vi "Create Missing Element.vi"(5 "Delimiter":string, 7 "Hierarchy":string[](array[string]), 10 "Element in":refnum<class "Config Element.lvclass">, 11 "Create":bool) -> (2 "Element":refnum<class "Config Element.lvclass">)   [LabVIEW 2020, in "CDM-Config.lvlib" / "Config Manager.lvclass"]
uses:
  Config Manager.lvclass
  Config Element/Config Element.lvclass
  <vilib>/AdvancedString/1D String Array to Delimited String.vi
  CDM-Config.lvlib
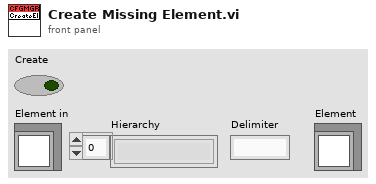
[diagram p1: front panel]
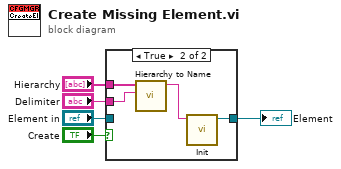
[diagram p0: block diagram]
diagram:
  n1 = case shown="True" "Create" {
    tunnel: "Element in" -> [w6 _]
    tunnel: [w6 w10] -> w3
    tunnel: "Delimiter" -> [_ w8]
    tunnel: "Hierarchy" -> [_ w9]
    frame False {
    }
    frame True {
      n2 = call "Hierarchy to Name.vi"("Delimiter"=w8, "Hierarchy"=w9) -> ("Full Name"=w7:string)  [unwired: 9 in]
      n3 = call "Init.vi"("Full Name"=w7) -> ("Config Element out"=w10:refnum<class "Config Element.lvclass">)  [unwired: 9 in, 1 out]
    }
  }
  "Element" <- w3
